vi "#4.vi"(0 "System no.":i32=1 min=1 max=4 step=1, 5 "error in":errorcluster) -> (14 "Status information":i32 format="%x", 15 "Status information (txt)":string, 19 "error out":errorcluster)   [LabVIEW 2020]
doc: "Request status information by sending the single ASCII character 4. Answer is controller specific. See controller user manual for decoding.\n\nC-887, F-206: Only for GCS syntax version = GCS 2.0 or higher (check with CSV?.vi. If CSV?.vi is not supported, syntax version is GCS 1.0).\n\nM-8X0: Only for controllers based on C-842.80 or GCS syntax version = GCS 2.0 or higher (Check with CSV?.vi. If CSV?.vi is not supported, syntax version is GCS 1.0)."
panel:
  # "Request status information."
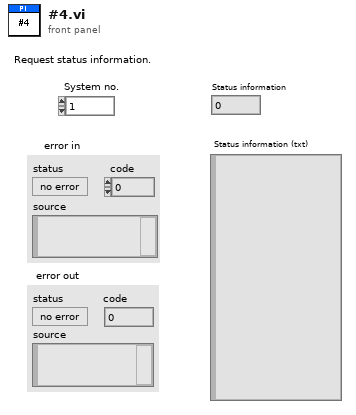
[diagram p1: front panel]
types:
  T1 = enum16{"Disable error check", "Force error check", "Use global settings"}
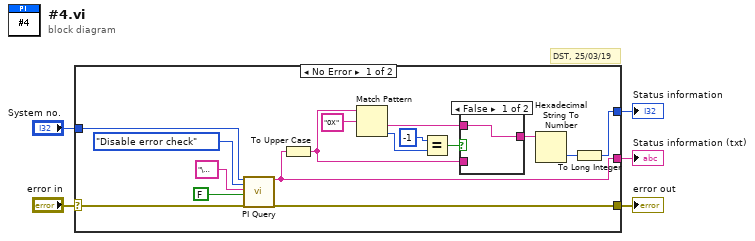
[diagram p0: block diagram]
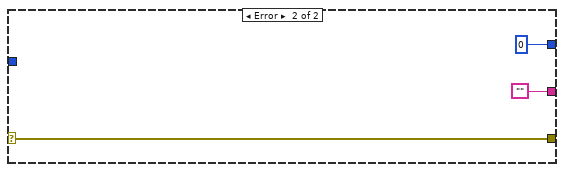
[diagram p3: hidden frame]
diagram:
  # "DST, 25/03/19"
  n1 = case shown="No Error" "error in" {
    selector: "error in" -> [w10 w25]
    tunnel: [w8 w25] -> w5
    tunnel: "System no." -> [w19 _]
    tunnel: [w9 "" ("String read")] -> w3
    tunnel: [w7 0] -> w1
    frame No Error {
      n2 = call "PI Query.vi"("System no."=w19, "Error check settings"=T1."Disable error check", "String to send"="\u0004", "Attach termination char.?"=FALSE ("Attach Linefeed?"), "error in"=w10) -> ("String read"=w9:string, "error out"=w8:errorcluster)  [unwired: 2 in, 11 out]
      n3 = To Upper Case(1:w9) -> (0:w11:string)
      n4 = Match Pattern(string=w11, regular expression="0X") -> (after substring=w13:string, offset past match=w16:i32)  [unwired: 3 out]
      n5 = Equal?(x=-1 ("y"), y=w16) -> (x = y?=w14:bool)
      n6 = case shown="False" w14 {
        tunnel: w11 -> [_ w23]
        tunnel: [w22 w23] -> w12
        tunnel: w13 -> [w22 _]
        frame False {
        }
        frame True {
        }
      }
      n7 = Hexadecimal String To Number(string=w12) -> (number=w18:u32)  [unwired: 3 out]
      n8 = To Long Integer(number=w18) -> (32bit integer=w7:i32)
    }
    frame Error {
    }
  }
  "error out" <- w5
  "Status information (txt)" <- w3
  "Status information" <- w1
